vi "Decode_TextFiles.vi"(8 "error in":errorcluster, 10 "Array":string[](array[string])) -> (0 "error out":errorcluster, 1 "Params":dbl[](array[numeric]), 2 "Signal":dbl[](array[numeric]), 3 "m/z list":dbl[](array[numeric]))   [LabVIEW 2012]
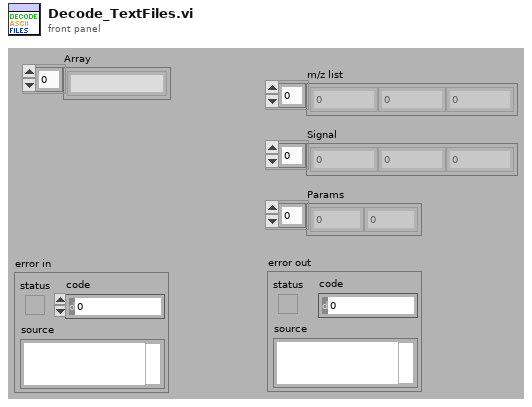
[diagram p1: front panel]
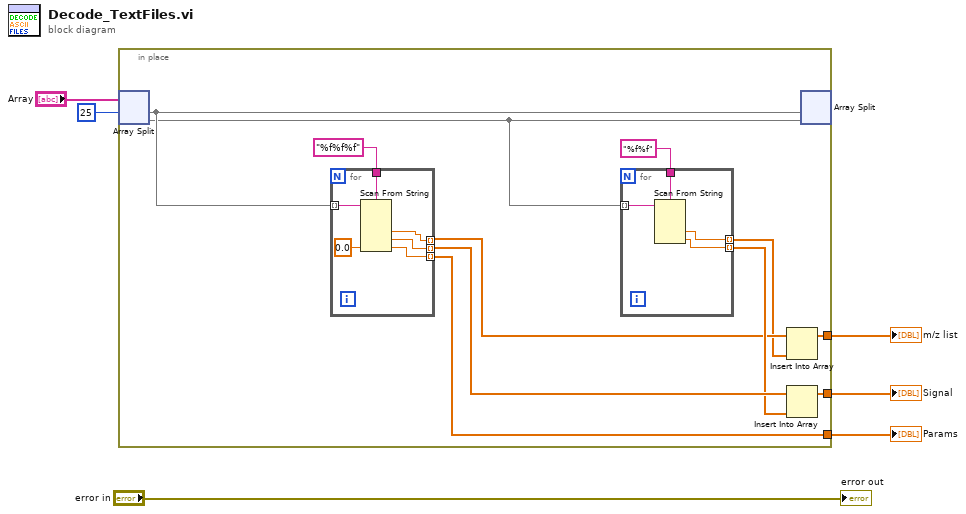
[diagram p0: block diagram]
diagram:
  n1 = in-place {
    in-place-border: [w17] -> w6
    in-place-border: [w14] -> w3
    in-place-border: [w9] -> w2
    n2 = in-place-split #1("Array", 25 ("index")) -> (w8:string[], w7:string[])
    n3 = for {
      tunnel: [w23] -> w17 mode=indexing
      tunnel: [w24] -> w13 mode=indexing
      tunnel: "%f%f%f" ("format string") -> [w27]
      tunnel: w8 -> [w26] mode=indexing
      tunnel: [w25] -> w11 mode=indexing
      n4 = Scan From String(format string=w27, input string=w26, default 3=0.0 ("default value 3")) -> (output 1=w25:dbl, output 2=w24:dbl, output 3=w23:dbl)  [unwired: 4 in, 3 out]
    }
    n5 = for {
      tunnel: [w18] -> w12 mode=indexing
      tunnel: "%f%f" ("format string") -> [w21]
      tunnel: w7 -> [w20] mode=indexing
      tunnel: [w19] -> w10 mode=indexing
      n6 = Scan From String(format string=w21, input string=w20) -> (output 1=w19:dbl, output 2=w18:dbl)  [unwired: 4 in, 3 out]
    }
    n7 = Insert Into Array(array=w11, new element=w10) -> (w9:dbl[])  [unwired: 1 in]
    n8 = Insert Into Array(array=w13, new element=w12) -> (w14:dbl[])  [unwired: 1 in]
    n9 = in-place-split #1(w8, w7) -> ()  [unwired: 2 out]
  }
  "Params" <- w6
  "Signal" <- w3
  "m/z list" <- w2
  "error out" <- "error in"
